vi "mlink_dio_write.vi"(8 "error in (no error)":errorcluster, 9 "state":bool, 10 "pin":u8, 11 "connection ID":i32=-1) -> (0 "error out":errorcluster, 3 "connection ID out":i32)   [LabVIEW 2009, in "MicroDAQ.lvlib" / "mlink.lvlib"]
uses:
  <instrlib>/MicroDAQ/Mlink library wraper/mlink.lvlib
  <instrlib>/MicroDAQ/MLink32.dll
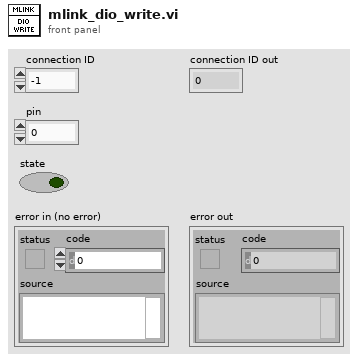
[diagram p1: front panel]
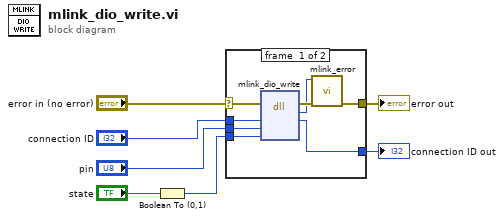
[diagram p0: block diagram]
diagram:
  n1 = Boolean To (0,1)(Boolean="state") -> (0, 1=w3:i16)
  n2 = case shown="No Error" "error in (no error)" {
    selector: "error in (no error)" -> [w13 w17]
    tunnel: "connection ID" -> [w15 w16]
    tunnel: [w14 w16] -> w6
    tunnel: w3 -> [w12 _]
    tunnel: "pin" -> [w11 _]
    tunnel: [w8 w17] -> w1
    frame #0 {
      n3 = dll-call lib="C:/Program Files (x86)/National Instruments/LabVIEW 2009/instr.lib/MicroDAQ/MLink32.dll" fn="mlink_dio_write"(error in=w13, "connection ID"=w15, "pin"=w11, "value"=w12) -> (error out=w10:errorcluster, "return type"=w9:i32, "connection ID"=w14:i32)  [unwired: 4 in, 1 out]
      n4 = call <instrlib>:"mlink_error.vi"("error in (no error)"=w10, "error code"=w9) -> ("error out"=w8:errorcluster)  [unwired: 9 in]
    }
    frame #1 {
    }
  }
  "connection ID out" <- w6
  "error out" <- w1
